vi "readFromXML.vi"(8 "error in (no error)":errorcluster, 10 "XML in":string, 11 "POffset in":refnum<class "POffset.lvclass">) -> (0 "error out":errorcluster, 3 "POffset out":refnum<class "POffset.lvclass">)   [LabVIEW 2014, in "TCSDataDefinitions.lvlib" / "TCSCommand.lvlib" / "POriginCommands.lvlib" / "POffset.lvclass"]
uses:
  POffset.lvclass
  OffsetCommands/OffsetDef/Enumerations/Num1Types.ctl
  <userlib>/Common/UnitsAndXML/FlattenItemWithUnitToXML/FlattenLengthToXML/LengthUnit.ctl
  POffset.lvclass/POffset.ctl
  POriginCommands/POriginCommands.lvclass
  <userlib>/Common/UnitsAndXML/UnitsAndXML.lvlib
  <userlib>/Common/XML/XMLParser/XMLParser.lvclass
  OffsetCommands/OffsetCommands.lvlib
panel:
  out "num1":T1
  out "dY":dbl[unit]
  out "dX":dbl[unit]
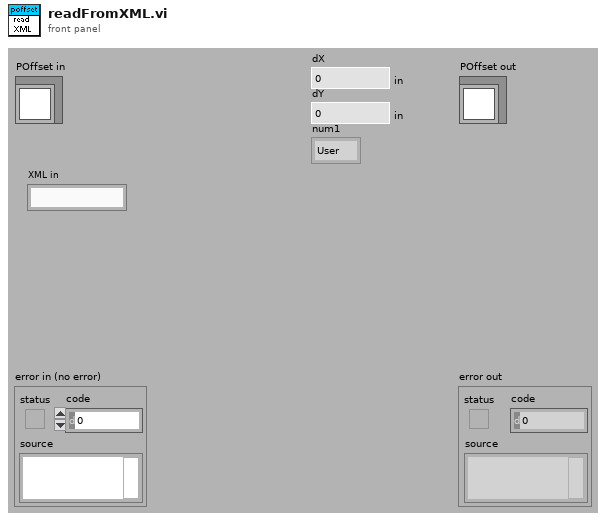
[diagram p1: front panel]
types:
  T1 = typedef "TCSDataDefinitions.lvlib/TCSCommand.lvlib/OffsetCommands.lvlib/Num1Types.ctl" = enum16{"User", "Handset"}
  T2 = typedef "UnitsAndXML.lvlib/LengthUnit.ctl" = enum16{"m", "Angstrom", "AU", "chain", "cm", "cubit", "fathom", "fermi", "ft", "furlong", "hubble", "in", "ly", "mi", "mm", "rod", "um", "yd"}
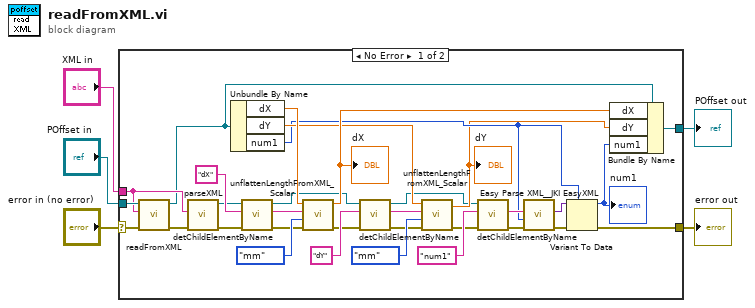
[diagram p0: block diagram]
diagram:
  n1 = case shown="No Error" "error in (no error)" {
    selector: "error in (no error)" -> [w34 w39]
    tunnel: [w10 w39] -> w4
    tunnel: [w30 w38] -> w2
    tunnel: "POffset in" -> [w32 w38]
    tunnel: "XML in" -> [w31 _]
    frame No Error {
      n2 = call-parent "readFromXML.vi"("error in (no error)"=w34, "XML in"=w31, "POriginCommands in"=w32) -> ("error out"=w33:errorcluster, "POriginCommands out"=w29:refnum<class "POffset.lvclass">)  [unwired: 7 out]
      n3 = call <userlib>:"parseXML.vi"("error in (no error)"=w33, "XMLString in"=w31) -> ("error out"=w35:errorcluster, "Element out"=w9:refnum<class "XMLParser.lvclass">)  [unwired: 8 in]
      n4 = Unbundle By Name(w29) -> ("dX"=w27:dbl[unit], "dY"=w21:dbl[unit], "num1"=w14:T1)
      n5 = call <userlib>:"detChildElementByName.vi"("error in (no error)"=w35, "childName"="dX" ("ChildName"), "Element in"=w9) -> ("error out"=w6:errorcluster, "childXML"=w26:string, "Element out"=w8:refnum<class "XMLParser.lvclass">)  [unwired: 5 in, 1 out]
      n6 = call <userlib>:"unflattenLengthFromXML_Scalar.vi"("error in (no error)"=w6, "lengthUnitInXML"=LengthUnit."mm", "xmlString"=w26, "lengthForType"=w27) -> ("error out"=w20:errorcluster, "length"=w24:dbl[unit])  [unwired: 6 in]
      "dX" <- w24
      n7 = call <userlib>:"detChildElementByName.vi"("error in (no error)"=w20, "childName"="dY" ("ChildName"), "Element in"=w8) -> ("error out"=w19:errorcluster, "childXML"=w22:string, "Element out"=w7:refnum<class "XMLParser.lvclass">)  [unwired: 5 in, 1 out]
      n8 = call <userlib>:"unflattenLengthFromXML_Scalar.vi"("error in (no error)"=w19, "lengthUnitInXML"=LengthUnit."mm", "xmlString"=w22, "lengthForType"=w21) -> ("error out"=w18:errorcluster, "length"=w12:dbl[unit])  [unwired: 6 in]
      "dY" <- w12
      n9 = call <userlib>:"detChildElementByName.vi"("error in (no error)"=w18, "childName"="num1" ("ChildName"), "Element in"=w7) -> ("error out"=w11:errorcluster, "childXML"=w15:string)  [unwired: 5 in, 2 out]
      n10 = call <vilib>:"Easy Parse XML__JKI EasyXML.vi"("error in (no error)"=w11, "LabVIEW Data (Type)"=w14, "XML String"=w15) -> ("error out"=w17:errorcluster, "LabVIEW Data"=w16:variant)  [unwired: 7 in]
      n11 = Variant To Data(error in=w17, type=w14, Variant=w16) -> (data=w13:T1, error out=w10:errorcluster)
      "num1" <- w13
      n12 = Bundle By Name(cluster=w29, "dX"=w24, "dY"=w12, "num1"=w13) -> (w30:refnum<class "POffset.lvclass">)
    }
    frame Error {
    }
  }
  "error out" <- w4
  "POffset out" <- w2
